vi "ReadCalibrationsFromDB.vi"   [LabVIEW 2016]
uses:
  <vilib>/Rock Robotics/Network Tables/NT Read Numeric Array.vi
  Configurations.vi
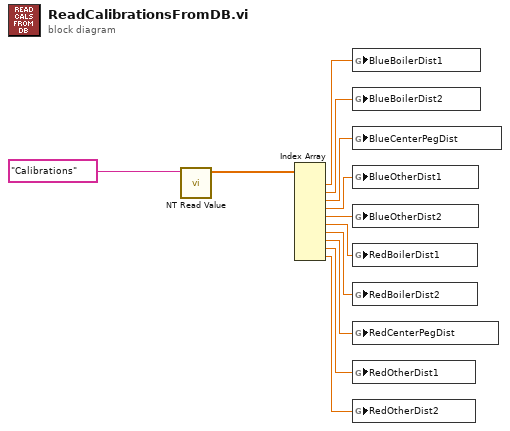
[diagram p0: block diagram]
diagram:
  n1 = call-poly <vilib>:"NT Read Value.vi"("Name"="Calibrations") -> ("Numeric Array"=w11:dbl[])  [unwired: 9 in, 1 out]
  n2 = Index Array(array=w11) -> (element #1=w10:dbl, element #2=w9:dbl, element #3=w8:dbl, element #4=w7:dbl, element #5=w6:dbl, element #6=w5:dbl, element #7=w4:dbl, element #8=w3:dbl, element #9=w2:dbl, element #10=w1:dbl)  [unwired: 10 in]
  n3 = global write "Configurations.vi" "BlueBoilerDist1"(w10) -> ()
  n4 = global write "Configurations.vi" "BlueBoilerDist2"(w9) -> ()
  n5 = global write "Configurations.vi" "BlueCenterPegDist"(w8) -> ()
  n6 = global write "Configurations.vi" "BlueOtherDist1"(w7) -> ()
  n7 = global write "Configurations.vi" "BlueOtherDist2"(w6) -> ()
  n8 = global write "Configurations.vi" "RedBoilerDist1"(w5) -> ()
  n9 = global write "Configurations.vi" "RedBoilerDist2"(w4) -> ()
  n10 = global write "Configurations.vi" "RedCenterPegDist"(w3) -> ()
  n11 = global write "Configurations.vi" "RedOtherDist1"(w2) -> ()
  n12 = global write "Configurations.vi" "RedOtherDist2"(w1) -> ()
